vi "Agilent 34970 Advanced Scan.vi"() -> ()   [LabVIEW 2012]
doc: "This example VI demonstrates setting up a scan list and taking a reading using the advanced VIs. For more information about the different types of VIs, see the descriptions below.\n\nEven though only two types of measurements are shown, all six types can be configured in the same way. Likewise, this VI does not show every available configurable option for voltage and resistance.\n\n====================\nSetting up and performing a scan\n====================\nThe HP34970A provides commands for setting up a scan in three ways that differ in their complexity and the amount of control offered:\n\n1. Advanced:\nEvery aspect of the measurement, scan, scan list, and read is put in a different command to allow the greatest flexibility. For example, using the advanced configure VIs, you can set up a scan list consisting of different measurement types on different channels. The \"HP34970A Advanced Scan Example.vi\" demonstrates usage of these VIs.\n\n2. Medium:\nThe instrument also offers a command that wraps up configuring individual channels and the scan list. This is represented in the driver by \"HP34970A Conf EZ.vi\". This driver specifically replaces use of the advanced configure measurement VIs and configure scan list VIs. For more information, refer to the context help for the Conf EZ VI.\n\n3. Easiest:\nThe entire configuration, scan, and read are wrapped up into one command to the instrument. This is provided in this driver as the \"EZ\" VIs, which are in the Data subpalette of the HP34970A's driver palette. The \"HP34970A EZ Scan Example.vi\" demonstrates the EZ VI's usage."
uses:
  <instrlib>/Agilent 34970/Agilent 34970.lvlib
panel:
  in  "Autorange (Res.)":bool
  in  "Autorange (Volt.)":bool
  in  "Serial Port Configuration":T1={"Timeout Value (10000)"=10000, "Baud Rate (57600)"=enum."57600", "Flow Control (1:XON/XOFF)"=enum."XON / XOFF"}
  in  "Reset (T: Reset)":bool=TRUE
  out "Readings":string[][](array[string])
  in  "4 Wire/2 Wire":bool
  in  "Range (Res.)":T2(ring)=enum."Maximum"
  in  "Channel List (Res.)":string
  in  "AC/DC":bool
  in  "Range (Volt.)":T3(ring)=enum."Maximum"
  in  "Channel List (Volt.)":string
  in  "Action":bool
  in  "VISA resource name":refnum<visa-resource-name>
  # "(c) 2005-2010 National Instruments.  ALL RIGHTS RESERVED."
  # "Voltage"
  # "Resistance"
  # "This example VI demonstrates setting up a scan list and taking a reading.  There are two ways to do that using this driver.  This method offers the most control.  Using the Configure VIs, you can create different types of readings in the same scan list.\n\nEven though only two types of measurements are shown, all six types can be configured in the same way."
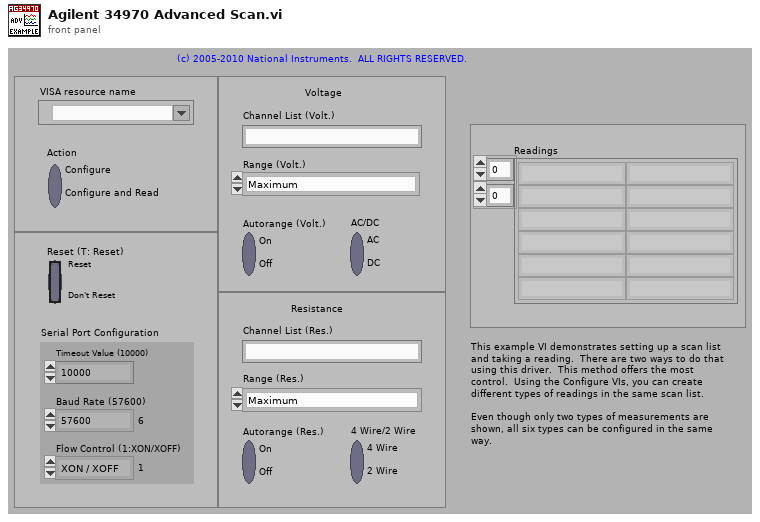
[diagram p1: front panel]
types:
  T1 = cluster{"Timeout Value (10000)":u32, "Baud Rate (57600)":enum16{"1200", "2400", "4800", "9600", "19200", "38400", "57600", "115200"}, "Flow Control (1:XON/XOFF)":enum16{"None", "XON / XOFF", "RTS / CTS", "DTR / DSR"}}
  T2 = enum16{"100 Ohm", "1 kOhm", "10 kOhm", "100 kOhm", "1 MOhm", "10 MOhm", "100 MOhm", "Minimum", "Maximum"}
  T3 = enum16{"100 mV", "1 V", "10 V", "100 V", "300 V", "Minimum", "Maximum"}
  T4 = cluster{"Include Alarm Data F:(No)":bool, "Include Channel # (F:No)":bool, "Include Time (F:No)":bool, "Include Units (F:No)":bool}
  T5 = enum16{"Enable Register", "Event Register", "Operation Complete Bit"}
  T6 = enum16{"Manual", "Minimum", "Maximum", "Infinity"}
  T7 = enum16{"Bus", "Immediate", "External", "Alarm 1", "Alarm 2", "Alarm 3", "Alarm 4", "Timer"}
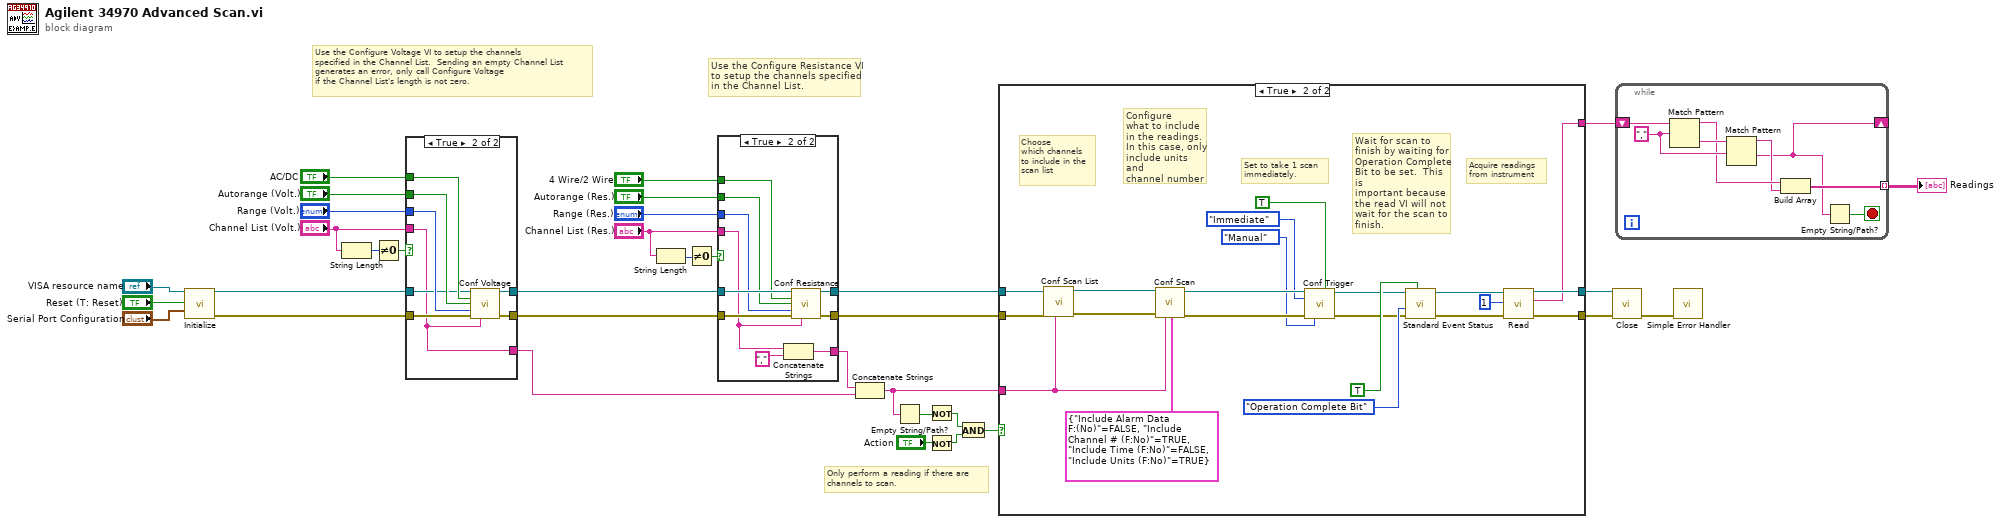
[diagram p0: block diagram]
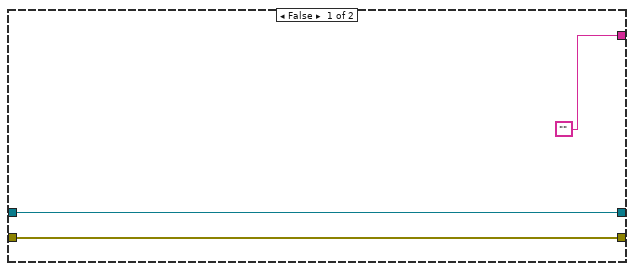
[diagram p2: hidden frame]
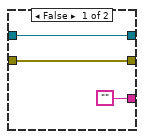
[diagram p3: hidden frame]
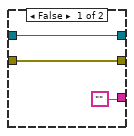
[diagram p4: hidden frame]
diagram:
  # "Only perform a reading if there are\nchannels to scan."
  # "Use the Configure Resistance VI\nto setup the channels specified\nin the Channel List."
  # "Use the Configure Voltage VI to setup the channels\nspecified in the Channel List.  Sending an empty Channel List\ngenerates an error, only call Configure Voltage\nif the Channel List's length is not zero."
  n1 = call <instrlib>:"Initialize.vi"("VISA Resource Name"="VISA resource name", "Reset (T: Reset)"="Reset (T: Reset)", "Serial Port Configuration"="Serial Port Configuration") -> ("VISA Resource Name Out"=w22:refnum<visa-resource-name>, "error out"=w21:errorcluster)  [unwired: 11 in]
  n2 = String Length(string="Channel List (Volt.)") -> (length=w28:i32)
  n3 = Not Equal To 0?(x=w28) -> (x != 0?=w27:bool)
  n4 = case shown="True" w27 {
    tunnel: "Channel List (Volt.)" -> [_ w38]
    tunnel: "Range (Volt.)" -> [_ w45]
    tunnel: "Autorange (Volt.)" -> [_ w44]
    tunnel: "AC/DC" -> [_ w43]
    tunnel: w22 -> [w37 w42]
    tunnel: w21 -> [w36 w41]
    tunnel: [w37 w40] -> w14
    tunnel: [w36 w39] -> w13
    tunnel: ["" w38] -> w9
    frame False {
    }
    frame True {
      n5 = call <instrlib>:"Conf Voltage.vi"("VISA Resource Name"=w42, "AC/DC (F:DC)"=w43, "Autorange? (F:Off)"=w44, "Range (6:Max)"=w45, "error in (no error)"=w41, "Channel List (empty)"=w38) -> ("VISA Resource Name Out"=w40:refnum<visa-resource-name>, "error out"=w39:errorcluster)  [unwired: 7 in, 1 out]
    }
  }
  n6 = String Length(string="Channel List (Res.)") -> (length=w19:i32)
  n7 = Not Equal To 0?(x=w19) -> (x != 0?=w20:bool)
  n8 = case shown="True" w20 {
    tunnel: "Channel List (Res.)" -> [_ w49]
    tunnel: "Range (Res.)" -> [_ w54]
    tunnel: "Autorange (Res.)" -> [_ w53]
    tunnel: "4 Wire/2 Wire" -> [_ w52]
    tunnel: w14 -> [w48 w58]
    tunnel: w13 -> [w47 w56]
    tunnel: [w48 w57] -> w12
    tunnel: [w47 w55] -> w11
    tunnel: ["" w51] -> w10
    frame False {
    }
    frame True {
      n9 = Concatenate Strings(w49, ",") -> (w51:string)
      n10 = call <instrlib>:"Conf Resistance.vi"("VISA Resource Name"=w58, "4 Wire/2 Wire (F:2)"=w52, "Autorange? (F:OFF)"=w53, "Range (8:Maximum)"=w54, "error in (no error)"=w56, "Channel List (empty)"=w49) -> ("VISA Resource Name Out"=w57:refnum<visa-resource-name>, "error out"=w55:errorcluster)  [unwired: 7 in, 1 out]
    }
  }
  n11 = Concatenate Strings(w10, w9) -> (w3:string)
  n12 = Empty String/Path?(string/path=w3) -> (empty?=w2:bool)
  n13 = Not(x=w2) -> (.not. x?=w1:bool)
  n14 = Not(x="Action") -> (.not. x?=w4:bool)
  n15 = And(x=w1, y=w4) -> (x .and. y?=w8:bool)
  n16 = case shown="True" w8 {
    tunnel: [w61 w65] -> w31
    tunnel: [w60 w66] -> w30
    tunnel: w12 -> [w61 w74]
    tunnel: w11 -> [w60 w73]
    tunnel: ["" w64] -> w7
    tunnel: w3 -> [_ w72]
    frame False {
    }
    frame True {
      # "Acquire readings\nfrom instrument"
      # "Wait for scan to \nfinish by waiting for \nOperation Complete \nBit to be set.  This is\nimportant because\nthe read VI will not \nwait for the scan to\nfinish."
      # "Set to take 1 scan\nimmediately."
      # "Configure\nwhat to include\nin the readings.\nIn this case, only\ninclude units and \nchannel number"
      # "Choose \nwhich channels\nto include in the\nscan list"
      n17 = call <instrlib>:"Conf Scan List.vi"("Scan List (empty)"=w72, "error in (no error)"=w73, "VISA Resource Name"=w74) -> ("error out"=w82:errorcluster, "VISA Resource Name Out"=w67:refnum<visa-resource-name>)  [unwired: 6 in, 1 out]
      n18 = call <instrlib>:"Conf Scan.vi"("VISA Resource Name"=w67, "error in (no error)"=w82, "Channel List (empty)"=w72, "Scan Fields"=T4 {"Include Alarm Data F:(No)"=FALSE, "Include Channel # (F:No)"=TRUE, "Include Time (F:No)"=FALSE, "Include Units (F:No)"=TRUE}) -> ("VISA Resource Name Out"=w80:refnum<visa-resource-name>, "error out"=w79:errorcluster)  [unwired: 9 in, 1 out]
      n19 = call <instrlib>:"Conf Trigger.vi"("VISA Resource Name"=w80, "Wait for Trigger? (F:No)"=TRUE, "Source (1:Immediate)"=T7."Immediate", "error in (no error)"=w79, "Max Trigger Count (3:Inf)"=T6."Manual") -> ("VISA Resource Name Out"=w63:refnum<visa-resource-name>, "error out"=w62:errorcluster)  [unwired: 8 in, 1 out]
      n20 = call <instrlib>:"Standard Event Status.vi"("Set/Check? (F:Set)"=TRUE, "error in (no error)"=w62, "Check Parameter (0:Enable Reg)"=T5."Operation Complete Bit", "VISA Resource Name"=w63) -> ("error out"=w75:errorcluster, "VISA Resource Name Out"=w76:refnum<visa-resource-name>)  [unwired: 5 in, 1 out]
      n21 = call <instrlib>:"Read.vi"("error in (no error)"=w75, "# Channels (1)"=1 ("# Channels (0)"), "VISA Resource Name"=w76) -> ("error out"=w66:errorcluster, "Readings"=w64:string, "VISA Resource Name Out"=w65:refnum<visa-resource-name>)  [unwired: 5 in, 1 out]
    }
  }
  n22 = call <instrlib>:"Close.vi"("VISA Resource Name"=w31, "error in (no error)"=w30) -> ("error out"=w29:errorcluster)  [unwired: 13 in]
  n23 = while {
    tunnel: [w85] -> w6 mode=indexing
    shift-left: w7 -> [w90]
    shift-right: [w83] -> _
    stop <- w84 stop-if-true
    w88 = "," ("regular expression")
    n24 = Match Pattern(string=w90, regular expression=w88) -> (before substring=w87:string, after substring=w89:string)  [unwired: 1 in, 2 out]
    n25 = Match Pattern(string=w89, regular expression=w88) -> (before substring=w86:string, after substring=w83:string)  [unwired: 1 in, 2 out]
    n26 = Build Array(w87, w86) -> (w85:string[])
    n27 = Empty String/Path?(string/path=w83) -> (empty?=w84:bool)
  }
  "Readings" <- w6
  n28 = call <vilib>:"Simple Error Handler.vi"("error in (no error)"=w29) -> ()  [unwired: 4 in, 5 out]
